vi "mclust_ICL.vi"() -> ()   [LabVIEW 2014]
panel:
  in  "hcUse":string
  in  "hcModelNames":string[](array[string])=["VVV", "EEE", "VII", "EII"]
  in  "G":i32[](array[numeric])
  in  "Initialization":T1
  in  "modelNames":string[](array[string])
  out "d (number of column)":i32
  out "n (number of row)":i32
  in  "Data":dbl[][](array[numeric])
  # "hcUse: determines how to scale\ndata\npossible options\n\"VARS\", \"STD\", \"PCR\", \"PCS\",\n\"SPH\",\"SVD\""
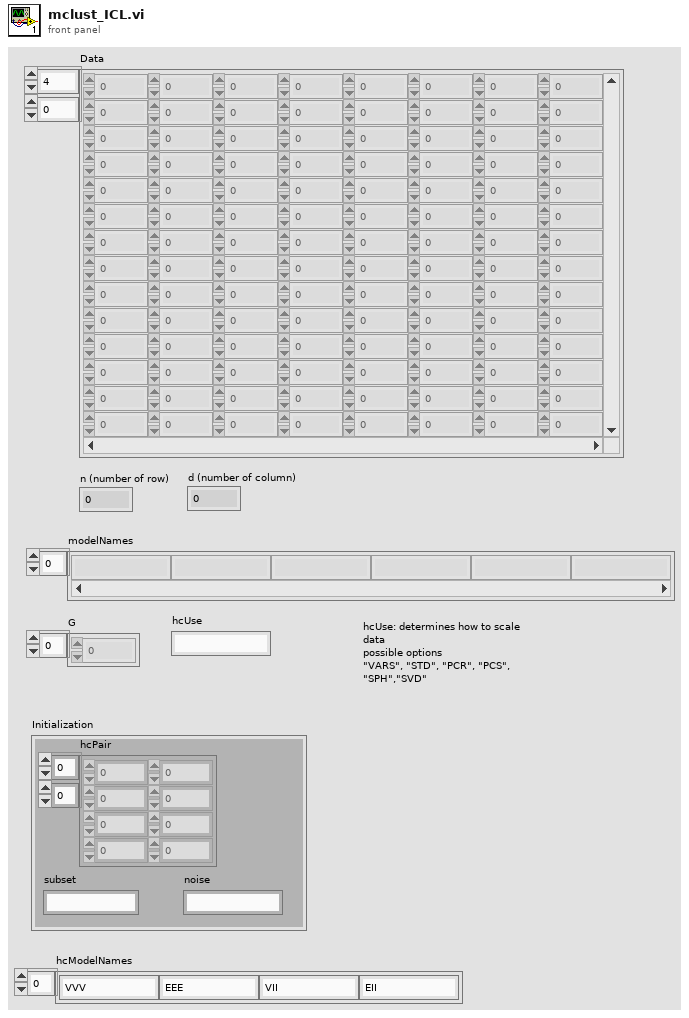
[diagram p1: front panel]
types:
  T1 = cluster{"subset":string, "noise":string, "hcPair":dbl[][]}
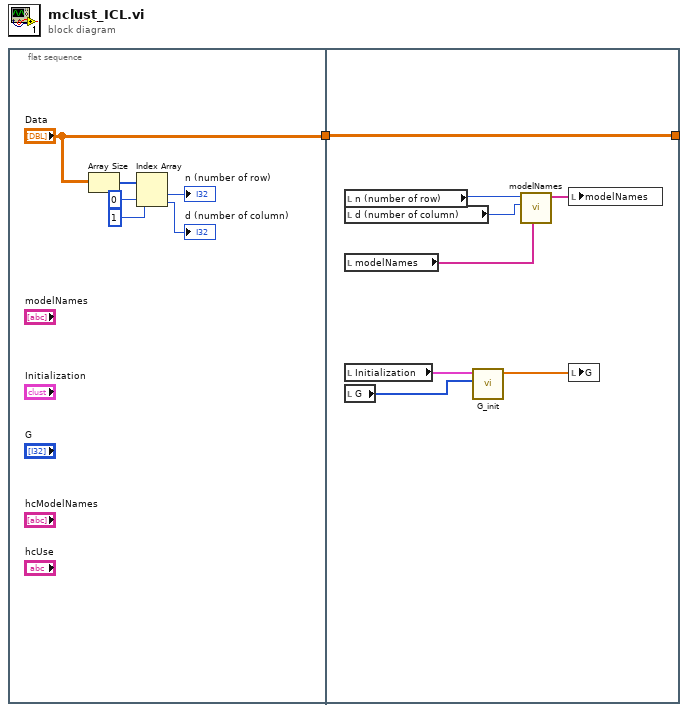
[diagram p0: block diagram]
diagram:
  n1 = flat-sequence {
    tunnel: ["Data"] -> w1
    tunnel: [w15] -> _
    tunnel: w1 -> [w15]
    frame #0 {
      n2 = Array Size(array="Data") -> (size(s)=w7:i32[])
      n3 = Index Array(array=w7, index #1=0 ("index"), index #2=1 ("index")) -> (element #1=→"n (number of row)":i32, element #2=→"d (number of column)":i32)
    }
    frame #1 {
      n4 = local read "n (number of row)"() -> (w14:i32)
      n5 = local read "d (number of column)"() -> (w13:i32)
      n6 = local read "modelNames"() -> (w12:string[])
      n7 = local read "Initialization"() -> (w8:T1)
      n8 = local read "G"() -> (w11:i32[])
      n9 = call "G_init.vi"("G"=w11, "Initialization"=w8) -> ("G(out)"=w10:dbl[])  [unwired: 9 in]
      n10 = call "modelNames.vi"("modelNames (in)"=w12, "d"=w13, "n"=w14) -> ("modelNames (out)"=w9:string[])  [unwired: 8 in]
      n11 = local write "modelNames"(w9) -> ()
      n12 = local write "G"(w10) -> ()
    }
  }
